vi "FlatToRichnixnet_grpc_J1939CommState.vi"(5 "OutputClusterType":T1, 11 "InputCluster":T2) -> (3 "OutputCluster":T1)   [LabVIEW 2025, in "grpc-xnet_client.lvlib"]
uses:
  grpc-xnet_client.lvlib
  nixnet_grpc_J1939CommState_Flat.ctl
  nixnet_grpc_J1939CommState.ctl
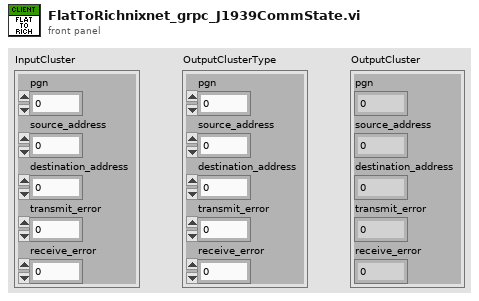
[diagram p1: front panel]
types:
  T1 = typedef "grpc-xnet_client.lvlib/nixnet_grpc_J1939CommState.ctl" = cluster{"pgn":u32, "source_address":u32, "destination_address":u32, "transmit_error":u32, "receive_error":u32}
  T2 = typedef "grpc-xnet_client.lvlib/nixnet_grpc_J1939CommState_Flat.ctl" = cluster{"pgn":u32, "source_address":u32, "destination_address":u32, "transmit_error":u32, "receive_error":u32}
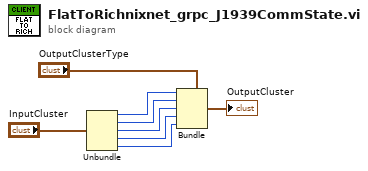
[diagram p0: block diagram]
diagram:
  n1 = Unbundle "Unbundle"("InputCluster") -> ("pgn"=w5:u32, "source_address"=w4:u32, "destination_address"=w3:u32, "transmit_error"=w2:u32, "receive_error"=w1:u32)
  n2 = Bundle "Bundle"(cluster="OutputClusterType", "pgn"=w5, "source_address"=w4, "destination_address"=w3, "transmit_error"=w2, "receive_error"=w1) -> (→"OutputCluster":T1)
